vi "Create.vi"(8 "error in (no error)":errorcluster, 10 "Input":string) -> (0 "error out":errorcluster, 3 "Map":refnum<class "Maze.lvclass">)   [LabVIEW 2021, in "Maze.lvclass"]
uses:
  Maze.lvclass
  Maze.lvclass/Maze.ctl
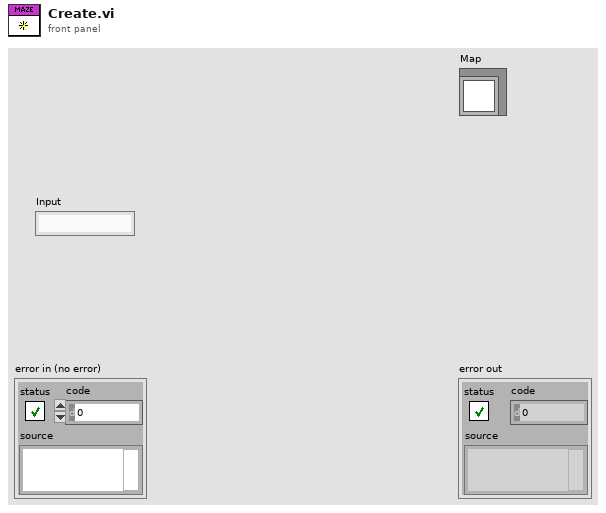
[diagram p1: front panel]
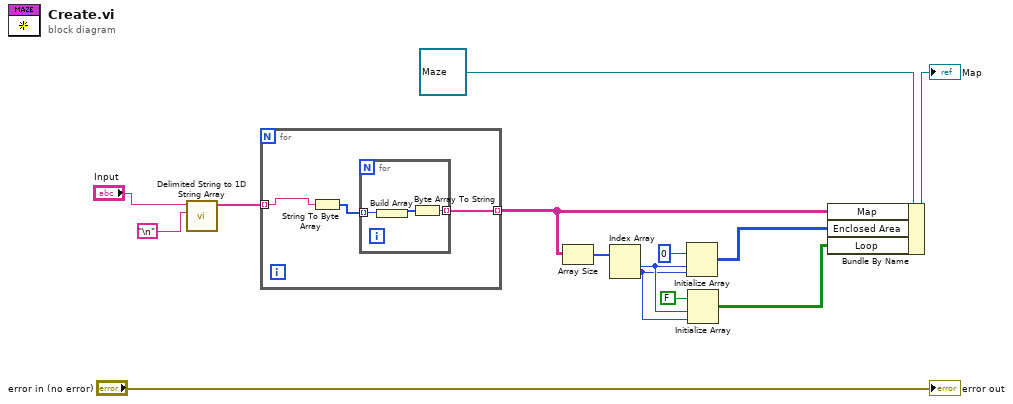
[diagram p0: block diagram]
diagram:
  n1 = call <vilib>:"Delimited String to 1D String Array.vi"("delimiter"="\n", "delimited string"="Input") -> ("string array"=w10:string[])  [unwired: 9 in]
  n2 = for {
    tunnel: w10 -> [w17] mode=indexing
    tunnel: [w15] -> w8 mode=indexing
    n3 = String To Byte Array(string=w17) -> (unsigned byte array=w16:u8[])
    n4 = for {
      tunnel: w16 -> [w20] mode=indexing
      tunnel: [w18] -> w15 mode=indexing
      n5 = Build Array(w20) -> (w19:u8[])
      n6 = Byte Array To String(unsigned byte array=w19) -> (string=w18:string)
    }
  }
  n7 = Array Size(array=w8) -> (size(s)=w7:i32[])
  n8 = Index Array(array=w7) -> (element #1=w4:i32, element #2=w3:i32)  [unwired: 2 in]
  n9 = Initialize Array(0 ("element"), w4, w3) -> (w5:i32[][])
  n10 = Initialize Array(FALSE, w4, w3) -> (w2:bool[][])
  n11 = Bundle By Name(cluster=refnum<class "Maze.lvclass"> refnum ("Map"), "Map"=w8, "Enclosed Area"=w5, "Loop"=w2) -> (→"Map":refnum<class "Maze.lvclass">)
  "error out" <- "error in (no error)"
